vi "Parse GPS Sentence.vi"   [LabVIEW 2017, in "NMEA API.lvlib"]
doc: "Returns data contained in a particular type of NMEA sentence. The input sentence you specify must include valid NMEA formatting and end with a carriage return and line feed, or \\r\\n. You must manually select the polymorphic instance to use."
uses:
  <vilib>/robotics/Protocols/NMEA/NMEA API.lvlib
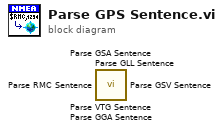
[diagram p0: block diagram]
diagram:
  n1 = call <vilib>:"Parse VTG Sentence.vi"() -> ()  [unwired: 10 in, 2 out]
  n2 = call <vilib>:"Parse GLL Sentence.vi"() -> ()  [unwired: 10 in, 2 out]
  n3 = call <vilib>:"Parse RMC Sentence.vi"() -> ()  [unwired: 10 in, 2 out]
  n4 = call <vilib>:"Parse GSV Sentence.vi"() -> ()  [unwired: 10 in, 2 out]
  n5 = call <vilib>:"Parse GGA Sentence.vi"() -> ()  [unwired: 10 in, 2 out]
  n6 = call <vilib>:"Parse GSA Sentence.vi"() -> ()  [unwired: 10 in, 2 out]
